vi "Extract2DArray.vi"() -> ()   [LabVIEW 2025]
panel:
  out "Waveform Graph 3":dbl[](graph)
  out "Waveform Graph 2":dbl[](graph)
  out "Waveform Graph":dbl[](graph)
  out "Array":dbl[][](array[numeric])
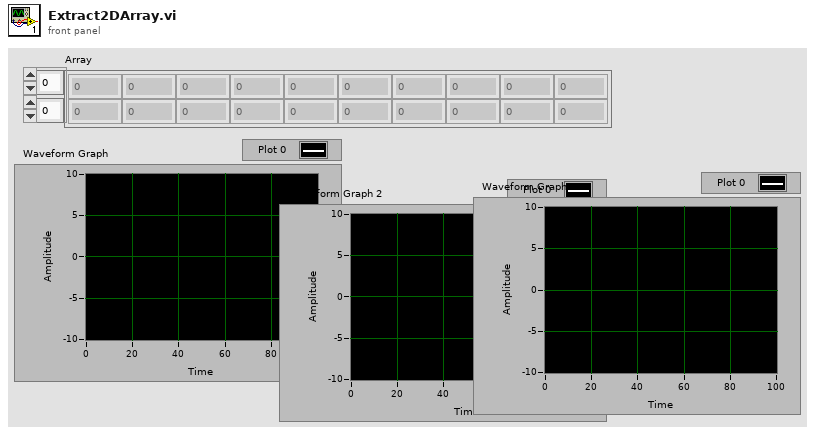
[diagram p1: front panel]
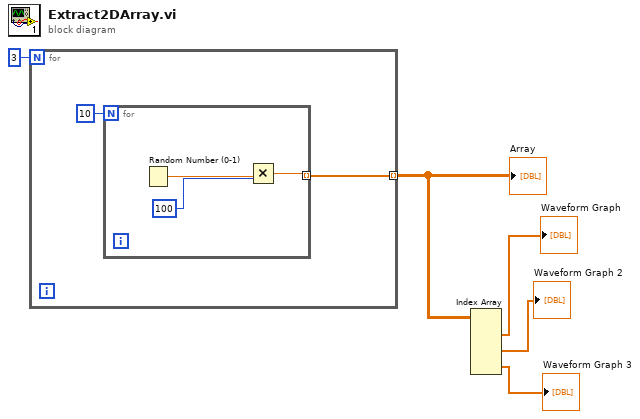
[diagram p0: block diagram]
diagram:
  n1 = for {
    N: 3 -> [_]
    tunnel: [w6] -> w4 mode=indexing
    n2 = for {
      N: 10 -> [_]
      tunnel: [w8] -> w6 mode=indexing
      n3 = Random Number (0-1)() -> (number: 0 to 1=w10:dbl)
      n4 = Multiply(x=w10, y=100) -> (x*y=w8:dbl)
    }
  }
  "Array" <- w4
  n5 = Index Array "Index Array"(array=w4) -> (element #1=→"Waveform Graph":dbl[], element #2=→"Waveform Graph 2":dbl[], element #3=→"Waveform Graph 3":dbl[])  [unwired: 6 in]
